vi "Configure Delay Time.vi"(0 "VISA resource name":refnum<visa-resource-name>, 5 "Delay (0.5 s)":dbl=0.5 min=0.5 max=999.9 format="%.1f", 11 "error in (no error)":errorcluster) -> (4 "VISA resource name out":refnum<visa-resource-name>, 15 "error out":errorcluster)   [LabVIEW 2020, in "eec 6700.lvlib"]
doc: "Sets the <B>Delay time</B> in the active memory of the power source instrument.\n\n<B>Range</B> : 0.1~999.9 s\n\nThe delay parameter configures a time delay, or warm up time. There is a voltage output present from the source, but the high and low limit thresholds are essentially ignored during this period."
uses:
  <instrlib>/eec 6700/eec 6700.lvlib
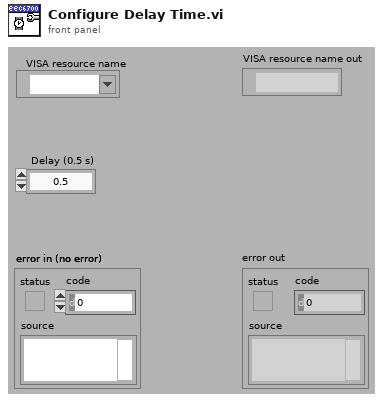
[diagram p1: front panel]
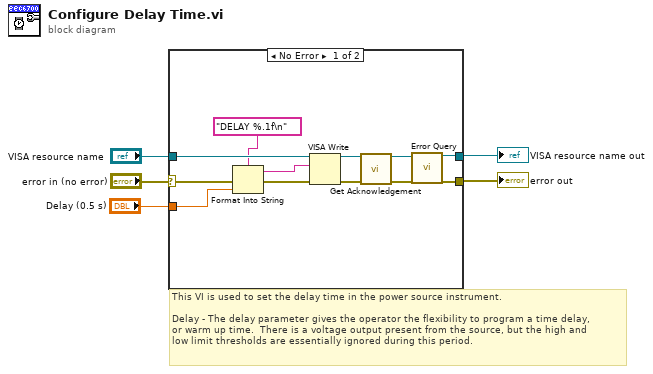
[diagram p0: block diagram]
diagram:
  # "This VI is used to set the delay time in the power source instrument.\n\nDelay - The delay parameter gives the operator the flexibility to program a time delay, \nor warm up time.  There is a voltage output present from the source, but the high and \nlow limit thresholds are essentially ignored during this period."
  n1 = case shown="No Error" "error in (no error)" {
    selector: "error in (no error)" -> [w11 w19]
    tunnel: "VISA resource name" -> [w17 w18]
    tunnel: [w13 w18] -> w4
    tunnel: [w12 w19] -> w3
    tunnel: "Delay (0.5 s)" -> [w16 _]
    frame No Error {
      n2 = Format Into String(format string="DELAY %.1f\n" ("Command"), error in=w11, w16) -> (resulting string=w15:string, error out=w10:errorcluster)  [unwired: 1 in]
      n3 = VISA Write(VISA resource name=w17, write buffer=w15, error in (no error)=w10) -> (VISA resource name out=w7:refnum<visa-resource-name>, error out=w6:errorcluster)  [unwired: 1 out]
      n4 = call <instrlib>:"Get Acknowledgement.vi"("VISA resource name"=w7, "error in (no error)"=w6) -> ("VISA resource name out"=w8:refnum<visa-resource-name>, "error out"=w9:errorcluster)  [unwired: 12 in]
      n5 = call <instrlib>:"Error Query.vi"("VISA resource name"=w8, "error in (no error)"=w9) -> ("VISA resource name out"=w13:refnum<visa-resource-name>, "error out"=w12:errorcluster)  [unwired: 10 in, 2 out]
    }
    frame Error {
    }
  }
  "error out" <- w3
  "VISA resource name out" <- w4
